vi "MPU6050 Read Rotation Data.vi"(8 "error in (no error)":errorcluster, 11 "I2C Ref In":T1={"myRIO Reference"={"myRIO Model"=enum."Unknown", "myRIO Hardware Reference"={"Generic FPGA Reference"=refnum, "Allow multiple opens"=FALSE}}, "I2C Channels Enum"=enum."Not Connected", "I2C Configuration"={"I2C Transfer Rate"=enum."Fast mode (400 kbps)"}}) -> (0 "error out":errorcluster, 2 "rad/s":cluster{"X":dbl, "Y":dbl, "Z":dbl}, 3 "Accel":cluster{dbl, dbl, dbl})   [LabVIEW 2018]
uses:
  <vilib>/myRIO/Instrument Drivers/Onboard IO/I2C/typedefs/I2C Reference.ctl
  <vilib>/myRIO/Common/Instrument Driver Framework/Utilities/typedefs/myRIO Generic Hardware Reference.ctl
  <vilib>/myRIO/Common/Instrument Driver Framework/Utilities/typedefs/Hardware Version Enum.ctl
  <vilib>/myRIO/Common/Instrument Driver Framework/Utilities/typedefs/myRIO v1.0 Reference.ctl
  <vilib>/myRIO/Common/Instrument Driver Framework/Utilities/typedefs/Generic FPGA Reference.ctl
  <vilib>/myRIO/Common/Instrument Driver Framework/myRIO v1.0/I2C/typedefs/I2C Channels Enum.ctl
  <vilib>/myRIO/Instrument Drivers/Onboard IO/I2C/typedefs/I2C Configuration.ctl
  <vilib>/myRIO/Instrument Drivers/Onboard IO/I2C/typedefs/I2C Transfer Rate.ctl
  MPU6050 Private class data.vi
  <vilib>/myRIO/Instrument Drivers/Onboard IO/I2C/I2C.lvlib
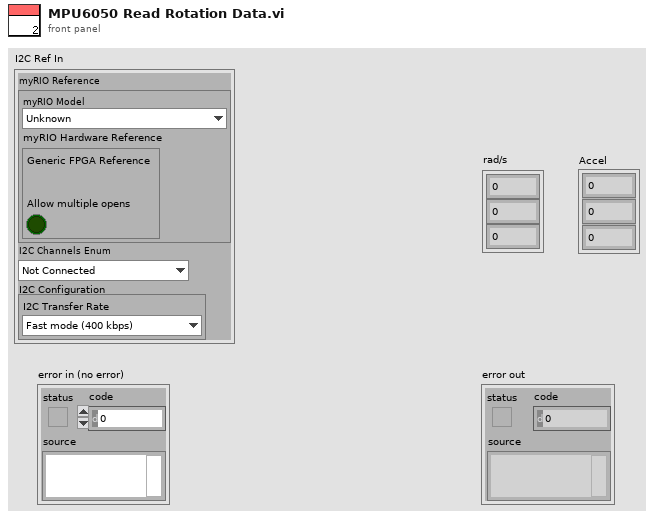
[diagram p1: front panel]
types:
  T1 = typedef "I2C.lvlib/I2C Reference.ctl" = cluster{"myRIO Reference":T2, "I2C Channels Enum":T6, "I2C Configuration":T7}
  T2 = typedef "myRIO Generic Hardware Reference.ctl" = cluster{"myRIO Model":T3, "myRIO Hardware Reference":T4}
  T3 = typedef "Hardware Version Enum.ctl" = enum16{"Unknown", "myRIO-1900", "myRIO-1950", "roboRIO", "NI ELVIS RIO CM", "ELVIS III"}
  T4 = typedef "myRIO v1.0 Reference.ctl" = cluster{"Generic FPGA Reference":T5, "Allow multiple opens":bool}
  T5 = typedef "Generic FPGA Reference.ctl" = refnum<k20>
  T6 = typedef "I2C Channels Enum.ctl" = enum16{"Not Connected", "A/I2C", "B/I2C", "I2C/I2C"}
  T7 = typedef "I2C.lvlib/I2C Configuration.ctl" = cluster{"I2C Transfer Rate":T8}
  T8 = typedef "I2C.lvlib/I2C Transfer Rate.ctl" = enum16{"Standard mode (100 kbps)", "Fast mode (400 kbps)"}
  T9 = cluster{"Data read[0]":u8, "Data read[1]":u8, "Data read[2]":u8, "Data read[3]":u8, "Data read[4]":u8, "Data read[5]":u8}
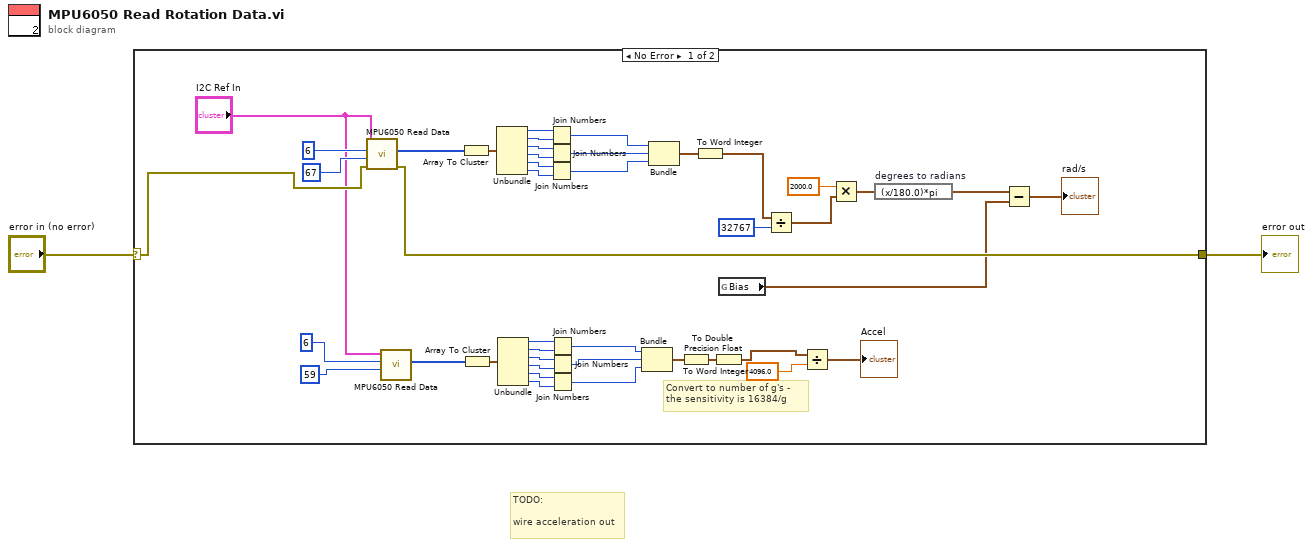
[diagram p0: block diagram]
diagram:
  # "TODO:\n\nwire acceleration out"
  n1 = case shown="No Error" "error in (no error)" {
    selector: "error in (no error)" -> [w23 w46]
    tunnel: [w24 w46] -> w1
    frame No Error {
      # "Convert to number of g's -\nthe sensitivity is 16384/g"
      n2 = call "MPU6050 Read Data.vi"("error in (no error)"=w23, "Start Address"=u8 67, "Data Length"=u8 6, "I2C Ref In"="I2C Ref In") -> ("error out"=w24:errorcluster, "Data read"=w42:u8[])  [unwired: 6 in]
      n3 = call "MPU6050 Read Data.vi"("Start Address"=u8 59, "Data Length"=u8 6, "I2C Ref In"="I2C Ref In") -> ("Data read"=w12:u8[])  [unwired: 7 in, 1 out]
      n4 = Array To Cluster(array=w42) -> (cluster=w41:T9)
      n5 = Array To Cluster(array=w12) -> (cluster=w13:T9)
      n6 = Unbundle(w41) -> ("Data read[0]"=w40:u8, "Data read[1]"=w39:u8, "Data read[2]"=w38:u8, "Data read[3]"=w37:u8, "Data read[4]"=w36:u8, "Data read[5]"=w35:u8)
      n7 = Unbundle(w13) -> ("Data read[0]"=w14:u8, "Data read[1]"=w15:u8, "Data read[2]"=w16:u8, "Data read[3]"=w17:u8, "Data read[4]"=w18:u8, "Data read[5]"=w19:u8)
      n8 = Join Numbers(hi=w40, lo=w39) -> ((hi.lo)=w45:u16)
      n9 = Join Numbers(hi=w38, lo=w37) -> ((hi.lo)=w44:u16)
      n10 = Join Numbers(hi=w36, lo=w35) -> ((hi.lo)=w43:u16)
      n11 = Join Numbers(hi=w14, lo=w15) -> ((hi.lo)=w11:u16)
      n12 = Join Numbers(hi=w16, lo=w17) -> ((hi.lo)=w10:u16)
      n13 = Join Numbers(hi=w18, lo=w19) -> ((hi.lo)=w9:u16)
      n14 = Bundle(w11, w10, w9) -> (w4:cluster{u16, u16, u16})  [unwired: 1 in]
      n15 = Bundle(w45, w44, w43) -> (w34:cluster{u16, u16, u16})  [unwired: 1 in]
      n16 = To Word Integer(number=w4) -> (16bit integer=w3:cluster{i16, i16, i16})
      n17 = To Word Integer(number=w34) -> (16bit integer=w27:cluster{i16, i16, i16})
      n18 = To Double Precision Float(number=w3) -> (double precision float=w8:cluster{dbl, dbl, dbl})
      n19 = global read "MPU6050 Private class data.vi" "Bias"() -> (w22:cluster{"X":dbl, "Y":dbl, "Z":dbl})
      n20 = Divide(x=w27, y=i16 32767) -> (x/y=w28:cluster{dbl, dbl, dbl})
      n21 = Divide(x=w8, y=4096.0) -> (x/y=→"Accel":cluster{dbl, dbl, dbl})
      n22 = Multiply(x=2000.0, y=w28) -> (x*y=w31:cluster{dbl, dbl, dbl})
      n23 = expression code="(x/180.0)*pi" "degrees to radians"(w31) -> (w25:cluster{dbl, dbl, dbl})
      n24 = Subtract(x=w25, y=w22) -> (x-y=→"rad/s":cluster{dbl, dbl, dbl})
    }
    frame Error {
    }
  }
  "error out" <- w1
